vi "libdaq_counter_get_ex.vi"(0 "error in (no error)":errorcluster, 1 "device_name":string, 2 "module_name":string) -> (14 "error out":errorcluster, 15 "device_name":string, 16 "module_name":string, 17 "period":u32, 18 "pulse":u32, 19 "count":u32)   [LabVIEW 2010, in "libdaqVI.lvlib"]
uses:
  libdaqVI.lvlib
  dll/daqlib.dll
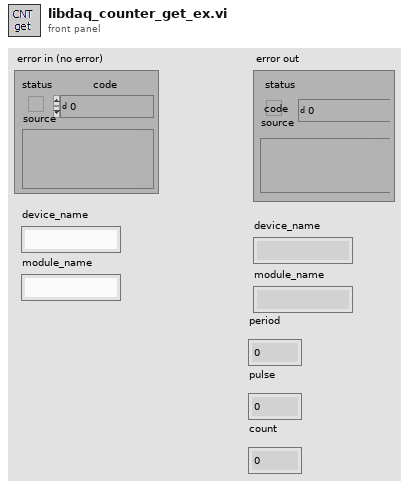
[diagram p1: front panel]
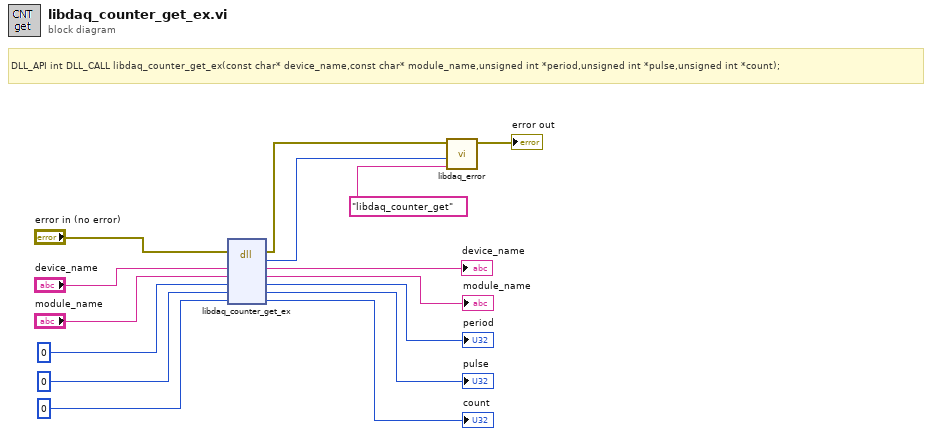
[diagram p0: block diagram]
diagram:
  # "DLL_API int DLL_CALL libdaq_counter_get_ex(const char* device_name,const char* module_name,unsigned int *period,unsigned int *pulse,unsigned int *count);"
  n1 = dll-call lib="E:/Product/Example/DAQ-USB3212/Labview/labview_2010/libdaqVI/dll/daqlib.dll" fn="libdaq_counter_get_ex"(error in="error in (no error)", "device_name"="device_name", "module_name"="module_name", "period"=0, "pulse"=0, "count"=0) -> (error out=w10:errorcluster, "return type"=w8:i32, "device_name"=→"device_name":string, "module_name"=→"module_name":string, "period"=→"period":u32, "pulse"=→"pulse":u32, "count"=→"count":u32)  [unwired: 2 in, 1 out]
  n2 = call "libdaq_error.vi"("error source"="libdaq_counter_get", "error code"=w8, "错误输入（无错误）"=w10) -> ("错误输出"=→"error out":errorcluster)  [unwired: 8 in]
